vi "mini_test_app_serial_gpib (capable of overlapping tests)_qmh_ver.vi"() -> ()   [LabVIEW 2015]
doc: "This template is for the Queued Message Handler design pattern.\n\nThe Event Handling Loop generates messages based on user interface actions.\n\nThe Message Handling Loop processes messages generated by the Event Handling Loop, or by other messages. The messages are string values, so new messages can be added easily to the Message Cases case structure in the Message Handling Loop. Each message cluster can also provide an optional value for Message Data, which is a variant that can be converted to whatever message-specific data is required."
uses:
  controls/UI Data.ctl
  controls/HP Data.ctl
  Type Definitions/Highway_GB_Data.ctl
  <vilib>/Utility/error.llb/Error Cluster From Error Code.vi
  support/Message Queue/Enqueue Message (Array).vi
  support/Message Queue/Enqueue Message (Single).vi
  <vilib>/ErrorRing/Error Ring.xnode
  support/Message Queue/Message Queue.lvlib
  support/User Event - Stop/User Event - Stop.lvlib
panel:
  out "tst mod":T1(ring) caption="Test mode"
  out "GB Display":string
  out "tst time":dbl caption="total test time"
  out "overlap":dbl
  out "2d tst":dbl caption="test time 2"
  out "1st tst":dbl caption="test time 1"
  out "delay":dbl caption="delay time"
  out "GB test":dbl(slide) scale=0.0..1.0 scale format="%#_3g"
  out "HP test":dbl(slide) caption="Hi-Pot test" scale=0.0..1.0 scale format="%#_3g"
  out "HP Display":string
  out "I/F type":string caption="Interface type"
  out "GB ID":string="\r\n" caption="GB Instrument ID"
  out "HP ID":string="\r\n" caption="Hi-Pot Instrument ID"
  out "GB tst reslts":string caption="GB test results"
  out "GB tst st":string caption="GB test status"
  out "HP tst rslts":string caption="Hi-Pot test results"
  out "HP tst st":string caption="Hi-Pot test status"
  out "Display <Replace Me>":string
  in  "Stop test":bool
  in  "Start test":bool
  in  "Exit Button":bool
  # "QMH version"
  # "Hi-Pot test"
  # "GB test"
  # "Warning. This app is a proof of concept and has no other purpose, \nit is not intended for production. Use at your own risk."
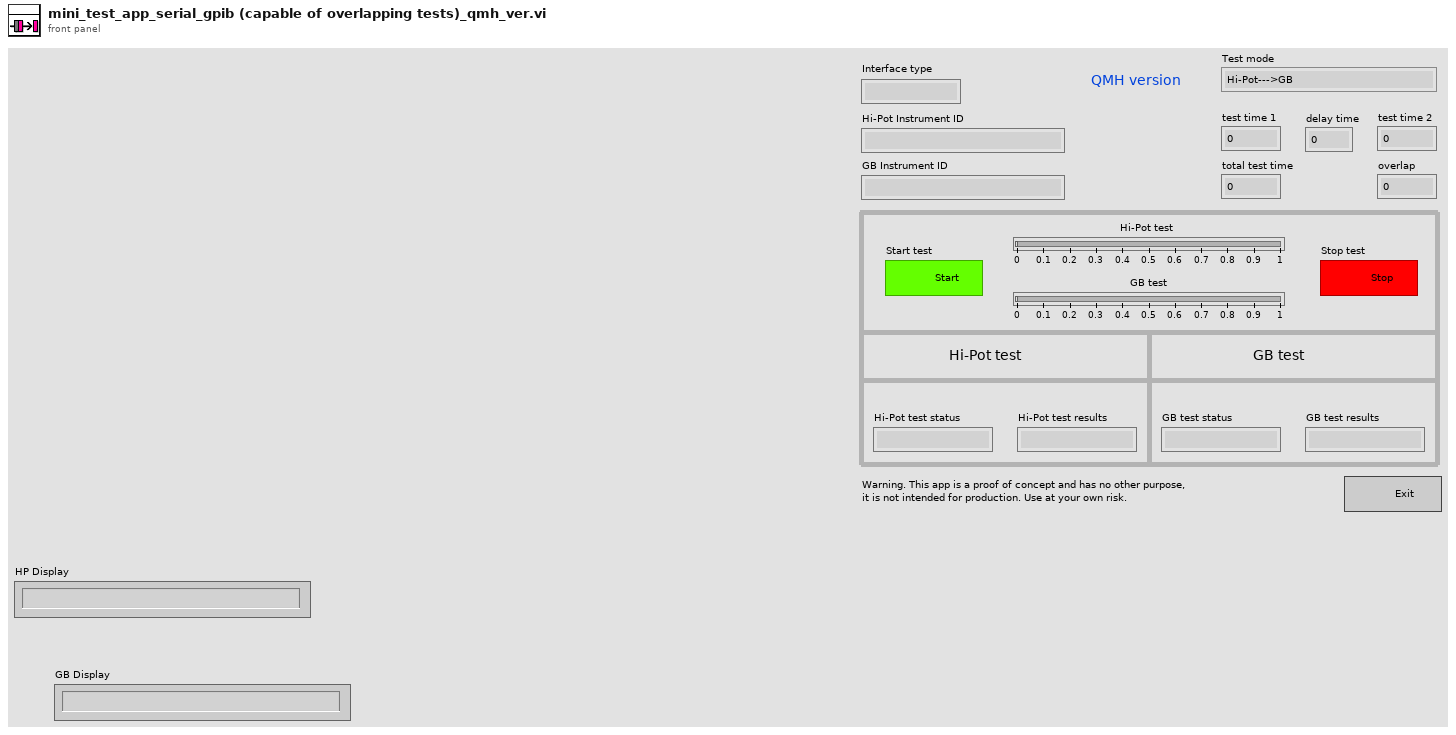
[diagram p1: front panel]
types:
  T1 = enum16{"Hi-Pot--->GB", "GB--->Hi-Pot", "Hi-Pot only", "GB only"}
  T2 = typedef "Highway_GB_Data.ctl" = cluster{"Status GB":string, "Results GB":string}
  T3 = typedef "HP Data.ctl" = cluster{"Status HP":string, "Results HP":string}
  T4 = typedef "UI Data.ctl" = cluster{"Delay Time":dbl, "prms":cluster{"1st tst":dbl, "2nd tst":dbl, "overlap":dbl, "tst time":dbl, "delay":dbl}, "test mode":enum16{"Hi-Pot--->GB", "GB--->Hi-Pot", "Hi-Pot only", "GB only"}}
  T5 = cluster{"test mode number":string, "test mode":enum16{"Hi-Pot--->GB", "GB--->Hi-Pot", "Hi-Pot only", "GB only"}, "size":i32}
  T6 = typedef "Rendezvous RefNum" = refnum<k1>
  T7 = cluster{"Rsrc name for 19572":refnum<visa-resource-name>, "Rsrc name for 19052":refnum<visa-resource-name>, "I/F type":string, "VISA2 Inst ID":string, "VISA1 Inst ID":string, "test mode":enum16{"Hi-Pot--->GB", "GB--->Hi-Pot", "Hi-Pot only", "GB only"}}
  T8 = typedef "Message Queue.lvlib/All Message Queues.ctl" = cluster{"Main":refnum<queue>, "GB Test":refnum<queue>, "HP Test":refnum<queue>}
  T9 = enum8{"Enabled", "Disabled", "Disabled and Grayed Out"}
  T10 = cluster{"1st tst":dbl, "2nd tst":dbl, "overlap":dbl, "tst time":dbl, "delay":dbl}
  T11 = cluster{"1st test":dbl, "2nd test":dbl, "overlap":dbl, "test time":dbl, "delay":dbl}
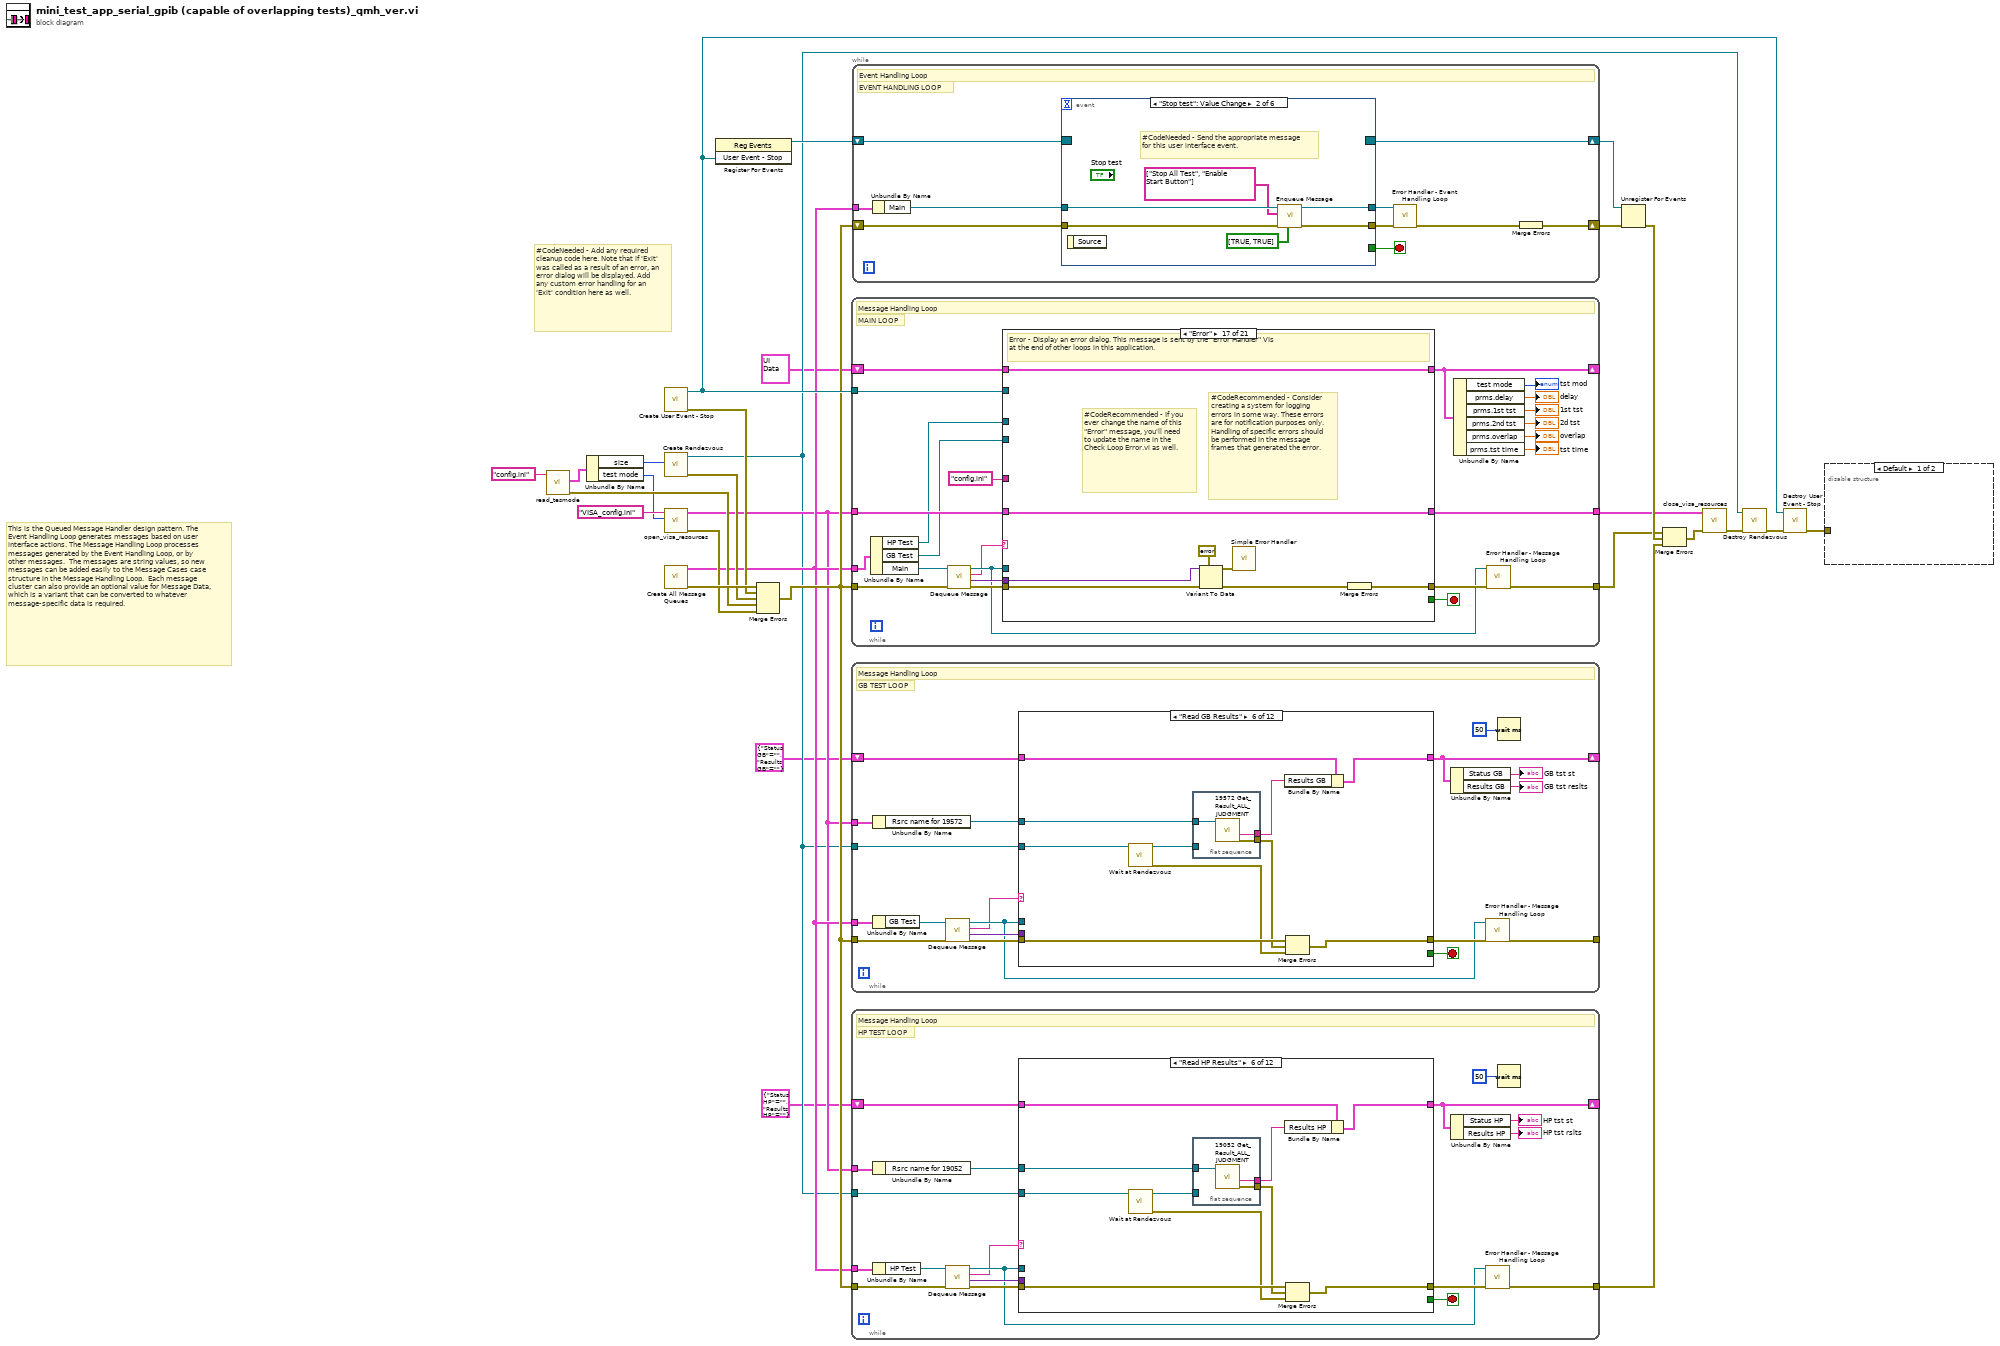
[diagram p0: block diagram]
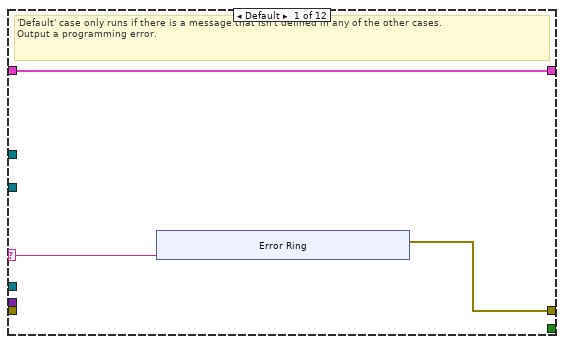
[diagram p2: hidden frame]
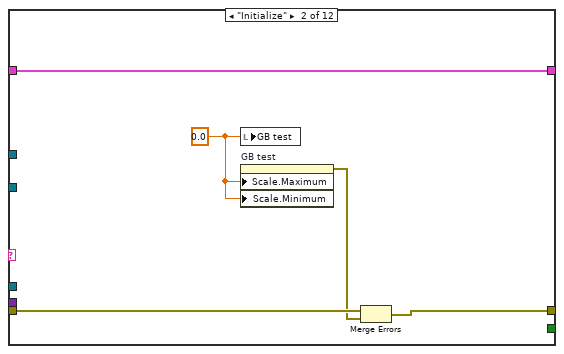
[diagram p3: hidden frame]
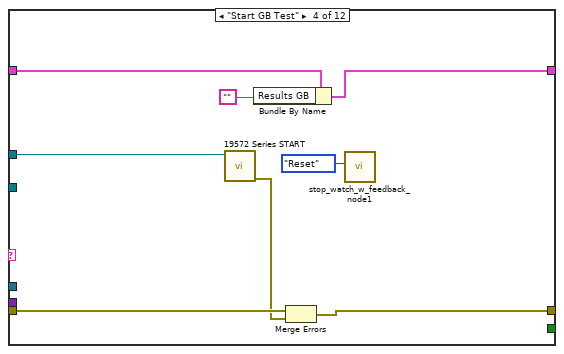
[diagram p5: hidden frame]
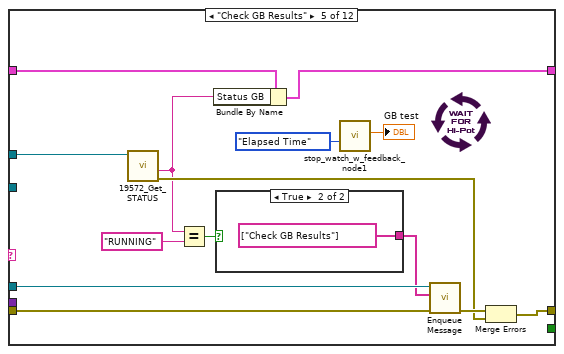
[diagram p6: hidden frame]
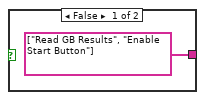
[diagram p7: hidden frame]
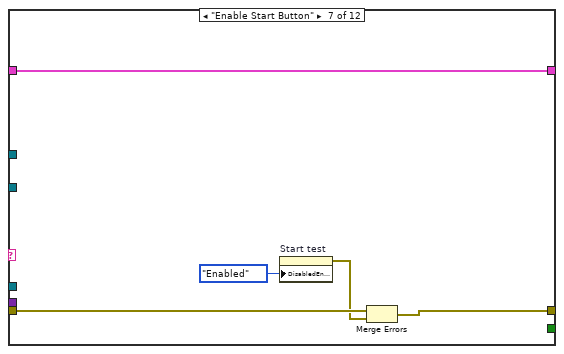
[diagram p8: hidden frame]
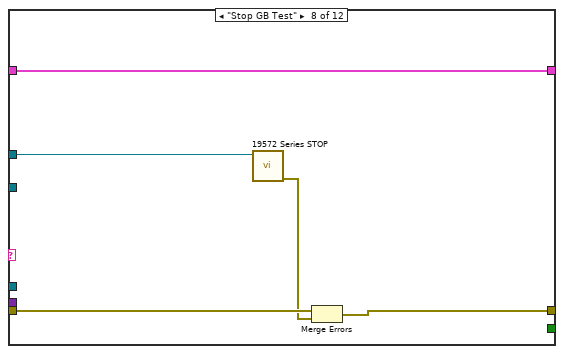
[diagram p9: hidden frame]
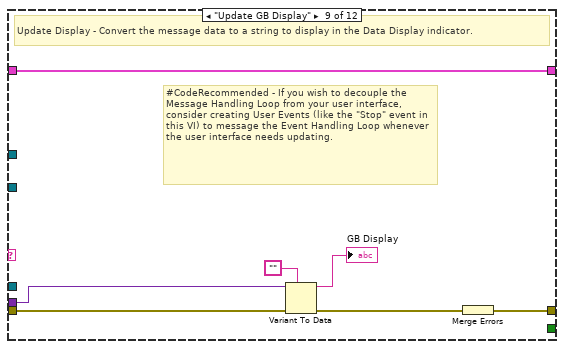
[diagram p10: hidden frame]
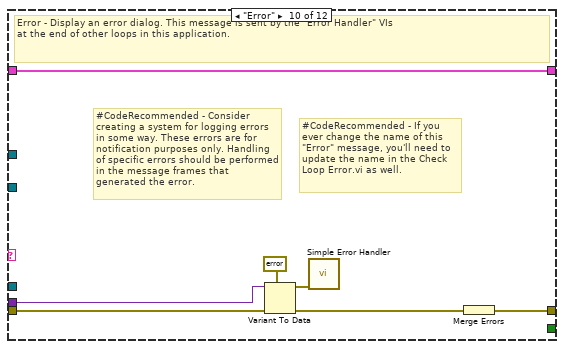
[diagram p11: hidden frame]
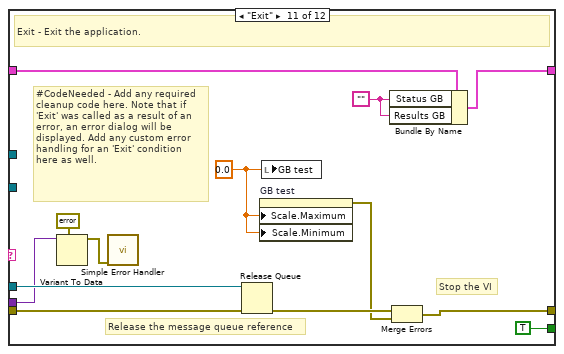
[diagram p12: hidden frame]
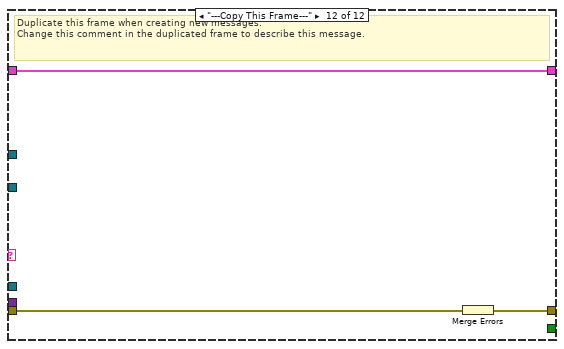
[diagram p13: hidden frame]
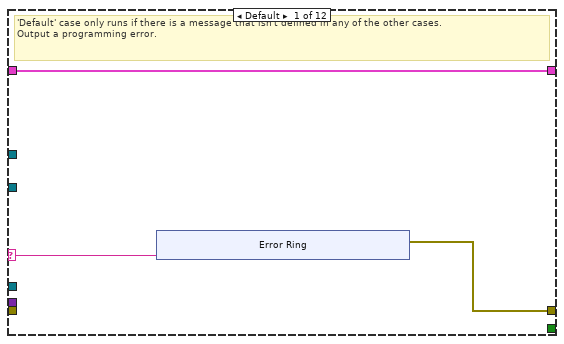
[diagram p14: hidden frame]
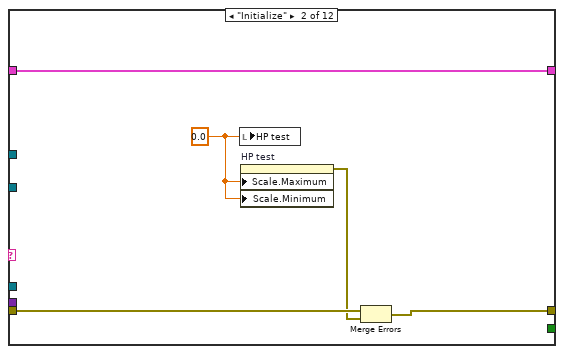
[diagram p15: hidden frame]
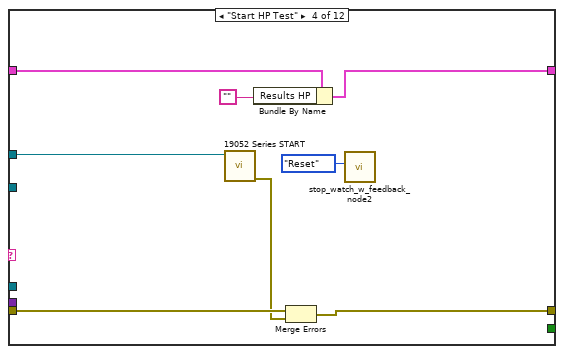
[diagram p17: hidden frame]
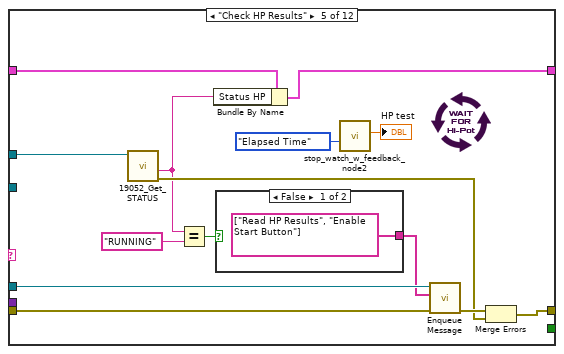
[diagram p18: hidden frame]
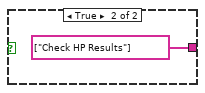
[diagram p19: hidden frame]
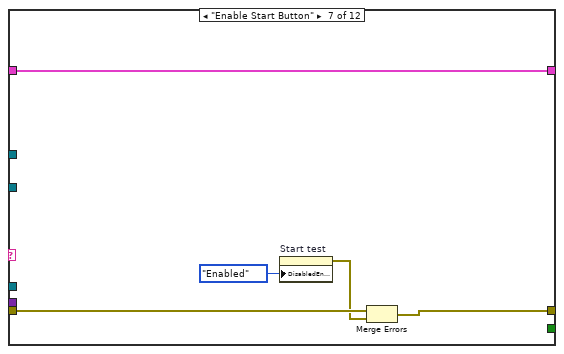
[diagram p20: hidden frame]
diagram:
  # "#CodeNeeded - Add any required cleanup code here. Note that if 'Exit' was called as a result of an error, an error dialog will be displayed. Add any custom error handling for an 'Exit' condition here as well."
  # "This is the Queued Message Handler design pattern. The Event Handling Loop generates messages based on user interface actions. The Message Handling Loop processes messages generated by the Event Handling Loop, or by other messages.  The messages are string values, so new messages can be added easily to the Message Cases case structure in the Message Handling Loop.  Each message cluster can also provide an optional value for Message Data, which is a variant that can be converted to whatever message-specific data is required."
  n1 = call "read_tesmode.vi"("config_file_name"="config.ini") -> ("error out"=w28:errorcluster, "test mode"=w6:T5)  [unwired: 8 in, 1 out]
  n2 = Unbundle By Name(w6) -> ("size"=w5:i32, "test mode"=w4:T1)
  n3 = call "Create User Event - Stop.vi"() -> ("error out"=w13:errorcluster, "User Event - Stop"=w12:refnum<user-event>)  [unwired: 10 in]
  n4 = call <vilib>:"Create Rendezvous.vi"("size (2)"=w5) -> ("error out"=w18:errorcluster, "rendezvous"=w8:T6)  [unwired: 4 in, 1 out]
  n5 = call "open_visa_resources.vi"("test mode"=w4, "config file in"="VISA_config.ini") -> ("error out"=w17:errorcluster, "VISA out"=w9:T7)  [unwired: 8 in]
  n6 = call "Create All Message Queues.vi"() -> ("error out"=w29:errorcluster, "Message Queues out"=w10:T8)  [unwired: 10 in]
  n7 = register-events(w12) -> (reference out=w24:refnum<event-registration>)  [unwired: 2 in, 1 out]
  n8 = Merge Errors(w29, w13, w18, w28, w17) -> (w11:errorcluster)
  n9 = while {
    shift-right: [w36] -> _
    shift-left: T4 {"Delay Time"=0.0, "prms"={"1st tst"=0.0, "2nd tst"=0.0, "overlap"=0.0, "tst time"=0.0, "delay"=0.0}, "test mode"=enum."Hi-Pot--->GB"} ("Data Cluster") -> [w52]
    tunnel: w12 -> [w51]
    tunnel: w11 -> [w50]
    tunnel: [w46] -> w21
    tunnel: w10 -> [w43]
    tunnel: w9 -> [w41]
    tunnel: [w40] -> w20
    stop <- w45 stop-if-true
    # "MAIN LOOP"
    # "Message Handling Loop"
    n10 = Unbundle By Name(w43) -> ("HP Test"=w39:refnum<queue>, "GB Test"=w38:refnum<queue>, "Main"=w42:refnum<queue>)
    n11 = call "Dequeue Message.vi"("error in (no error)"=w50, "Message Queue"=w42) -> ("error out"=w49:errorcluster, "Message Data"=w48:variant, "Message"=w44:string, "dup Message Queue"=w47:refnum<queue>)  [unwired: 6 in]
    n12 = case "Message Cases" shown="\"Error\"" w44 {
      selector: w44 -> [w55 _ _ _ _ _ _ _ _ _ _ _ _ _ _ _ _ _ _ _ _]
      tunnel: w47 -> [_ _ _ _ _ _ _ _ w129 _ _ _ _ _ _ _ _ w237 _ _ w270]
      tunnel: w49 -> [_ w71 w82 w92 w103 w115 w118 w124 w131 w142 w157 w171 w178 w194 w212 w218 w228 w241 w247 w255 w265]
      tunnel: [w56 w72 w81 w91 w102 w106 w118 w122 w132 w152 w167 w174 w181 w192 w208 w219 w222 w239 w245 w255 w267] -> w53
      tunnel: w52 -> [w57 w76 w80 w86 w95 w107 w117 w123 w127 w148 w163 w172 w179 w193 w211 w220 w227 w240 w246 w252 w269]
      tunnel: [w57 w76 w79 w85 w96 w107 w117 w123 w127 w148 w163 w172 w179 w193 w211 w220 w227 w240 w246 w251 w269] -> w36
      tunnel: [_ _ _ _ _ _ _ _ _ _ _ _ _ _ _ _ _ _ _ _ TRUE] -> w45
      tunnel: w48 -> [_ _ _ _ _ _ _ _ _ _ _ _ _ _ _ w217 w226 w232 _ _ w262]
      tunnel: w51 -> [_ _ _ _ _ _ _ _ _ _ _ _ _ _ _ _ _ _ _ _ w266]
      tunnel: w41 -> [w54 w74 w78 w90 w94 w114 w116 w121 w128 w151 w166 w173 w180 w187 w210 w213 w221 w236 w244 w254 w271]
      tunnel: [w54 w74 w78 w90 w94 w114 w116 w121 w128 w151 w166 w173 w180 w187 w210 w213 w221 w236 w244 w254 w271] -> w40
      tunnel: w39 -> [_ _ _ _ _ _ _ _ _ w143 w158 w168 _ w191 _ _ _ _ _ _ w258]
      tunnel: w38 -> [_ _ _ _ _ _ _ _ _ w144 w159 _ w175 w189 _ _ _ _ _ _ w257]
      tunnel: "config.ini" -> [_ _ _ w83 _ _ _ _ _ _ _ _ _ _ _ _ _ _ _ _ _]
      frame Default {
        # "'Default' case only runs if there is a message that isn't defined in any of the other cases. \nOutput a programming error."
        n13 = xnode "Error Ring"("parameter 0"=w55) -> ("error out"=w56:errorcluster)
      }
      frame "Initialize" {
        # "Bundle control references and a sample string value."
        # "Initialize - All initialization work should take place in this message, since other loops can potentially enqueue messages that execute immediately after this one."
        n14 = invoke on="Exit Button" class="Bool" method="Reinit To Default"() -> (error out=w69:errorcluster)  [unwired: 3 in, 2 out]
        n15 = invoke on="Stop test" class="Bool" method="Reinit To Default"() -> (error out=w70:errorcluster)  [unwired: 3 in, 2 out]
        n16 = Unbundle By Name(w74) -> ("VISA1 Inst ID"=→"GB ID":string, "VISA2 Inst ID"=→"HP ID":string, "I/F type"=→"I/F type":string)
        n17 = invoke on="Start test" class="Bool" method="Reinit To Default"(error in=w70) -> (error out=w68:errorcluster)  [unwired: 2 in, 2 out]
        n18 = property on="Start test" class="Bool"("DisabledEnum"=T9."Enabled" ("Disabled")) -> (error out=w67:errorcluster)  [unwired: 2 in, 1 out]
        n19 = Merge Errors(w71, w67, w69, w68) -> (w72:errorcluster)
      }
      frame "Get test mode" {
        # "Duplicate this frame when creating new messages.\nChange this comment in the duplicated frame to describe this message."
        n20 = Unbundle By Name(w78) -> ("test mode"=w77:T1)
        n21 = Merge Errors(w82) -> (w81:errorcluster)
        n22 = Bundle By Name(cluster=w80, "test mode"=w77) -> (w79:T4)
      }
      frame "Read delay time" {
        # "Duplicate this frame when creating new messages.\nChange this comment in the duplicated frame to describe this message."
        n23 = call "read_delay_time.vi"("config_file_name"=w83) -> ("error out"=w87:errorcluster, "values"=w88:cluster{"delay_time":string})  [unwired: 8 in, 1 out]
        n24 = call "delay_time_control.vi"("Higher limit"=100.0, "values in"=w88) -> ("delay time"=w84:dbl)  [unwired: 5 in]
        n25 = Merge Errors(w92, w87) -> (w91:errorcluster)
        n26 = Bundle By Name(cluster=w86, "Delay Time"=w84) -> (w85:T4)
      }
      frame "Read test params" {
        # "Duplicate this frame when creating new messages.\nChange this comment in the duplicated frame to describe this message."
        n27 = Unbundle By Name(w95) -> ("Delay Time"=w98:dbl, "test mode"=w97:T1)
        n28 = Unbundle By Name(w94) -> ("Rsrc name for 19052"=w99:refnum<visa-resource-name>, "Rsrc name for 19572"=w100:refnum<visa-resource-name>)
        n29 = call "test_definitions_module.vi"("Delay time"=w98, "VISA resource in 19572"=w100, "VISA resource in 19052"=w99, "test mode"=w97) -> ("error out"=w93:errorcluster, "Mode parameters"=w101:T11)  [unwired: 6 in]
        n30 = Bundle By Name(cluster=w95, "prms"=w101) -> (w96:T4)
        n31 = Merge Errors(w103, w93) -> (w102:errorcluster)
      }
      frame "Set Slides" {
        w113 = 0.0
        n32 = Unbundle By Name(w107) -> ("prms.1st tst"=w109:dbl, "prms.2nd tst"=w110:dbl, "test mode"=w108:T1)
        n33 = call "test_number_selector.vi"("1st tst in"=w109, "2nd tst in"=w110, "test mode"=w108) -> ("1st tst out"=w112:dbl, "2nd tst out"=w111:dbl)  [unwired: 2 in]
        n34 = property on="HP test" class="Slide (strict)"("Scale.Maximum"=w112, "Scale.Minimum"=w113) -> (error out=w104:errorcluster)  [unwired: 2 in, 1 out]
        n35 = property on="GB test" class="Slide (strict)"("Scale.Maximum"=w111, "Scale.Minimum"=w113) -> (error out=w105:errorcluster)  [unwired: 2 in, 1 out]
        n36 = Merge Errors(w115, w104, w105) -> (w106:errorcluster)
      }
      frame "Wait" {
      }
      frame "Disable Start Button" {
        # "Duplicate this frame when creating new messages.\nChange this comment in the duplicated frame to describe this message."
        n37 = property on="Start test" class="Bool"("DisabledEnum"=T9."Disabled and Grayed Out" ("Disabled")) -> (error out=w119:errorcluster)  [unwired: 2 in, 1 out]
        n38 = Merge Errors(w124, w119) -> (w122:errorcluster)
      }
      frame "Check Test Mode" {
        # "Send string to \"Update Display\" message"
        # "#CodeNeeded - Perform whatever actions correspond to the \"Something\" message."
        # "Something - Replace this message with functionality for your own application."
        n39 = Unbundle By Name(w127) -> ("test mode"=w126:T1)
        n40 = case shown="\"GB--->Hi-Pot\"" w126 {
          tunnel: ["Wait" "Start HP-->GB" "Start GB-->HP" "Start HP only" "Start GB only"] -> w125
          frame Default {
          }
          frame "Hi-Pot--->GB" {
          }
          frame "GB--->Hi-Pot" {
          }
          frame "Hi-Pot only" {
          }
          frame "GB only" {
          }
        }
        n41 = call-poly "Enqueue Message.vi"("error in (no error)"=w131, "Message"=w125, "Message Queue"=w129) -> ("error out"=w130:errorcluster)  [unwired: 7 in, 1 out]
        n42 = Merge Errors(w130) -> (w132:errorcluster)
      }
      frame "Start HP-->GB" {
        # "#CodeNeeded - Perform whatever actions correspond to the \"Something Else\" message."
        # "Something Else - Replace this message with functionality for your own application."
        n43 = call "select_queue_path.vi"("Control"=enum16{"Invert", "Direct"}."Invert", "Message Queue 2"=w144, "Message Queue"=w143) -> ("dup Message Queue 2"=w146:refnum<queue>, "dup Message Queue"=w145:refnum<queue>)  [unwired: 7 in]
        n44 = Unbundle By Name(w148) -> ("prms.delay"=w138:dbl)
        n45 = call-poly "Enqueue Message.vi"("Message Array"=string[] ["Start HP Test", "Check HP Results"], "Message Queue"=w146) -> ("error out"=w150:errorcluster)  [unwired: 8 in, 1 out]
        n46 = call "Time Delay"("error in (no error)"=w150, "Delay Time (s)"=w138) -> ("error out"=w149:errorcluster)  [unwired: 9 in]
        n47 = call-poly "Enqueue Message.vi"("error in (no error)"=w149, "Message Array"=string[] ["Start GB Test", "Check GB Results"], "Message Queue"=w145) -> ("error out"=w141:errorcluster)  [unwired: 7 in, 1 out]
        n48 = Merge Errors(w142, w141) -> (w152:errorcluster)
      }
      frame "Start GB-->HP" {
        # "#CodeNeeded - Perform whatever actions correspond to the \"Something Else\" message."
        # "Something Else - Replace this message with functionality for your own application."
        n49 = call "select_queue_path.vi"("Control"=enum16{"Invert", "Direct"}."Direct", "Message Queue 2"=w159, "Message Queue"=w158) -> ("dup Message Queue 2"=w161:refnum<queue>, "dup Message Queue"=w160:refnum<queue>)  [unwired: 7 in]
        n50 = Unbundle By Name(w163) -> ("prms.delay"=w153:dbl)
        n51 = call-poly "Enqueue Message.vi"("Message Array"=string[] ["Start GB Test", "Check GB Results"], "Message Queue"=w161) -> ("error out"=w165:errorcluster)  [unwired: 8 in, 1 out]
        n52 = call "Time Delay2"("error in (no error)"=w165, "Delay Time (s)"=w153) -> ("error out"=w164:errorcluster)  [unwired: 9 in]
        n53 = call-poly "Enqueue Message.vi"("error in (no error)"=w164, "Message Array"=string[] ["Start HP Test", "Check HP Results"], "Message Queue"=w160) -> ("error out"=w156:errorcluster)  [unwired: 7 in, 1 out]
        n54 = Merge Errors(w157, w156) -> (w167:errorcluster)
      }
      frame "Start HP only" {
        # "#CodeNeeded - Perform whatever actions correspond to the \"Something Else\" message."
        # "Something Else - Replace this message with functionality for your own application."
        n55 = call-poly "Enqueue Message.vi"("Message Array"=string[] ["Start HP Test", "Check HP Results"], "Message Queue"=w168) -> ("error out"=w170:errorcluster)  [unwired: 8 in, 1 out]
        n56 = Merge Errors(w171, w170) -> (w174:errorcluster)
      }
      frame "Start GB only" {
        # "#CodeNeeded - Perform whatever actions correspond to the \"Something Else\" message."
        # "Something Else - Replace this message with functionality for your own application."
        n57 = call-poly "Enqueue Message.vi"("Message Array"=string[] ["Start GB Test", "Check GB Results"], "Message Queue"=w175) -> ("error out"=w177:errorcluster)  [unwired: 8 in, 1 out]
        n58 = Merge Errors(w178, w177) -> (w181:errorcluster)
      }
      frame "Stop All Test" {
        n59 = Unbundle By Name(w187) -> ("test mode"=w186:T1)
        n60 = case shown="\"GB only\"" w186 {
          tunnel: w191 -> [w197 w202 w206]
          tunnel: [w197 w202 w206] -> w190
          tunnel: w189 -> [w196 w201 w205]
          tunnel: [w196 w201 w205] -> w188
          tunnel: ["Wait" "Stop GB Test" "Stop GB Test"] -> w185
          tunnel: ["Stop HP Test" "Stop HP Test" "Wait"] -> w184
          frame "Hi-Pot only" {
          }
          frame "Hi-Pot--->GB", "GB--->Hi-Pot" {
          }
          frame "GB only" {
          }
        }
        n61 = call-poly "Enqueue Message.vi"("Message"=w185, "Message Queue"=w188) -> ("error out"=w182:errorcluster)  [unwired: 8 in, 1 out]
        n62 = call-poly "Enqueue Message.vi"("Message"=w184, "Message Queue"=w190) -> ("error out"=w183:errorcluster)  [unwired: 8 in, 1 out]
        n63 = Merge Errors(w194, w183, w182) -> (w192:errorcluster)
      }
      frame "Enable Start Button" {
        n64 = property on="Start test" class="Bool"("DisabledEnum"=T9."Enabled" ("Disabled")) -> (error out=w207:errorcluster)  [unwired: 2 in, 1 out]
        n65 = Merge Errors(w212, w207) -> (w208:errorcluster)
      }
      frame "Update Display" {
        # "#CodeRecommended - If you wish to decouple the Message Handling Loop from your user interface, consider creating User Events (like the \"Stop\" event in this VI) to message the Event Handling Loop whenever the user interface needs updating."
        # "Update Display - Convert the message data to a string to display in the Data Display indicator."
        n66 = Variant To Data(error in=w218, type="", Variant=w217) -> (data=→"Display <Replace Me>":string, error out=w215:errorcluster)
        n67 = Merge Errors(w215) -> (w219:errorcluster)
      }
      frame "Error" {
        # "#CodeRecommended - If you ever change the name of this \"Error\" message, you'll need to update the name in the Check Loop Error.vi as well."
        # "#CodeRecommended - Consider creating a system for logging errors in some way. These errors are for notification purposes only. Handling of specific errors should be performed in the message frames that generated the error."
        # "Error - Display an error dialog. This message is sent by the \"Error Handler\" VIs \nat the end of other loops in this application."
        n68 = Variant To Data(error in=w228, type=errorcluster {"status"=FALSE, "code"=0, "source"=""} ("error constant"), Variant=w226) -> (data=w224:errorcluster, error out=w223:errorcluster)
        n69 = call <vilib>:"Simple Error Handler.vi"("error in (no error)"=w224) -> ()  [unwired: 4 in, 5 out]
        n70 = Merge Errors(w223) -> (w222:errorcluster)
      }
      frame "Confirm Quit" {
        # "#CodeNeeded - If you want to provide an \"Are you sure\" dialog (or some other notification) before the application exits, place that code here. This message is typically sent from a Panel Close? event."
        # "Confirm Quit - Message that can confirm whether or not the user wants to exit the application."
        n71 = Variant To Data(type="", Variant=w232) -> (data=w231:string, error out=w230:errorcluster)  [unwired: 1 in]
        n72 = Two Button Dialog(message=w231) -> (T button?=w235:bool)  [unwired: 2 in]
        n73 = case shown="True" w235 {
          tunnel: [string[] ["Wait"] string[] ["Exit", "Turn Off Indicators"]] -> w229
          frame False {
          }
          frame True {
          }
        }
        n74 = call-poly "Enqueue Message.vi"("Priority Message? Array"=bool[] [TRUE, TRUE], "error in (no error)"=w241, "Message Array"=w229, "Message Queue"=w237) -> ("error out"=w238:errorcluster)  [unwired: 6 in, 1 out]
        n75 = Merge Errors(w238, w230) -> (w239:errorcluster)
      }
      frame "---Copy This Frame---" {
        # "Duplicate this frame when creating new messages. Change this comment in the duplicated frame to describe this message."
        n76 = Merge Errors(w247) -> (w245:errorcluster)
      }
      frame "Turn Off Indicators" {
        w250 = ""
        n77 = local write "I/F type"(w250) -> ()
        n78 = local write "HP ID"(w250) -> ()
        n79 = local write "GB ID"(w250) -> ()
        n80 = Bundle By Name(cluster=w252, "test mode"=T1."Hi-Pot only", "Delay Time"=0.0, "prms"=T10 {"1st tst"=0.0, "2nd tst"=0.0, "overlap"=0.0, "tst time"=0.0, "delay"=0.0}) -> (w251:T4)
      }
      frame "Exit" {
        # "Stop the VI"
        # "Release the message queue reference"
        # "Exit - Exit the application."
        n81 = Variant To Data(type=errorcluster {"status"=FALSE, "code"=0, "source"=""} ("error constant"), Variant=w262) -> (data=w263:errorcluster)  [unwired: 1 in, 1 out]
        n82 = call <vilib>:"Simple Error Handler.vi"("error in (no error)"=w263) -> ()  [unwired: 4 in, 5 out]
        n83 = Unbundle By Name(w271) -> ("test mode"=w256:T1)
        n84 = Release Queue(queue=w270, error in (no error)=w265) -> (error out=w261:errorcluster)  [unwired: 1 in, 2 out]
        n85 = call "exit-tasks.vi"("test mode"=w256, "GB Test Queue"=w257, "HP Test Queue"=w258) -> ("error out"=w259:errorcluster)  [unwired: 8 in]
        n86 = call "Fire User Event - Stop.vi"("User Event - Stop"=w266) -> ("error out"=w260:errorcluster)  [unwired: 10 in]
        n87 = Merge Errors(w261, w260, w259) -> (w267:errorcluster)
      }
    }
    n88 = Unbundle By Name(w36) -> ("test mode"=→"tst mod":T1, "prms.delay"=→"delay":dbl, "prms.1st tst"=→"1st tst":dbl, "prms.2nd tst"=→"2d tst":dbl, "prms.overlap"=→"overlap":dbl, "prms.tst time"=→"tst time":dbl)
    n89 = call "Error Handler - Message Handling Loop.vi"("error in (no error)"=w53, "Message Queue"=w47) -> ("dup error in"=w46:errorcluster)  [unwired: 8 in, 1 out]
  }
  n90 = while {
    shift-right: [w279] -> _
    shift-left: T2 {"Status GB"="", "Results GB"=""} ("Data Cluster") -> [w288]
    tunnel: w11 -> [w287]
    tunnel: [w283] -> _
    tunnel: w9 -> [w281]
    tunnel: w10 -> [w277]
    tunnel: w8 -> [w275]
    stop <- w282 stop-if-true
    # "GB TEST LOOP"
    # "Message Handling Loop"
    n91 = Unbundle By Name(w281) -> ("Rsrc name for 19572"=w280:refnum<visa-resource-name>)
    n92 = Unbundle By Name(w277) -> ("GB Test"=w276:refnum<queue>)
    n93 = call "Dequeue Message.vi"("error in (no error)"=w287, "Message Queue"=w276) -> ("error out"=w286:errorcluster, "Message Data"=w285:variant, "Message"=w274:string, "dup Message Queue"=w284:refnum<queue>)  [unwired: 6 in]
    n94 = case "Message Cases" shown="\"Read GB Results\"" w274 {
      selector: w274 -> [w290 _ _ _ _ _ _ _ _ _ _ _]
      tunnel: w284 -> [_ _ _ _ w325 _ _ _ _ _ w380 _]
      tunnel: w286 -> [_ w302 w306 w313 w327 w340 w348 w350 w358 w367 w376 w383]
      tunnel: [w291 w301 w306 w312 w328 w339 w345 w352 w359 w361 w377 w381] -> w289
      tunnel: w288 -> [w292 w304 w305 w309 w323 w336 w347 w353 w360 w366 w370 w382]
      tunnel: [w292 w304 w305 w308 w322 w335 w347 w353 w360 w366 w369 w382] -> w279
      tunnel: [_ _ _ _ _ _ _ _ _ _ TRUE _] -> w282
      tunnel: w285 -> [_ _ _ _ _ _ _ _ w357 w365 w373 _]
      tunnel: w280 -> [_ _ _ w314 w324 w338 _ w351 _ _ _ _]
      tunnel: w275 -> [_ _ _ _ _ w331 _ _ _ _ _ _]
      frame Default {
        # "'Default' case only runs if there is a message that isn't defined in any of the other cases. \nOutput a programming error."
        n95 = xnode "Error Ring"("parameter 0"=w290) -> ("error out"=w291:errorcluster)
      }
      frame "Initialize" {
        w303 = 0.0
        n96 = local write "GB test"(w303) -> ()
        n97 = property on="GB test" class="Slide (strict)"("Scale.Maximum"=w303, "Scale.Minimum"=w303) -> (error out=w300:errorcluster)  [unwired: 2 in, 1 out]
        n98 = Merge Errors(w302, w300) -> (w301:errorcluster)
      }
      frame "Wait" {
      }
      frame "Start GB Test" {
        n99 = call "19572 Series START.vi"("VISA resource in"=w314) -> ("error out"=w311:errorcluster)  [unwired: 9 in, 1 out]
        n100 = Bundle By Name(cluster=w309, "Results GB"="") -> (w308:T2)
        n101 = Merge Errors(w313, w311) -> (w312:errorcluster)
        n102 = call "stop_watch_w_feedback_node1.vi"("Command"=enum16{"Elapsed Time", "Reset"}."Reset") -> ()  [unwired: 10 in, 1 out]
      }
      frame "Check GB Results" {
        n103 = call "19572_Get_STATUS.vi"("VISA resource in"=w324) -> ("error out"=w318:errorcluster, "Status"=w317:string)  [unwired: 8 in, 1 out]
        n104 = Equal?(x=w317, y="RUNNING") -> (x = y?=w320:bool)
        n105 = Bundle By Name(cluster=w323, "Status GB"=w317) -> (w322:T2)
        n106 = case shown="True" w320 {
          tunnel: [string[] ["Read GB Results", "Enable Start Button"] string[] ["Check GB Results"]] -> w319
          frame False {
          }
          frame True {
          }
        }
        n107 = call "stop_watch_w_feedback_node1.vi"("Command"=enum16{"Elapsed Time", "Reset"}."Elapsed Time") -> ("Elapsed Time"=→"GB test":dbl)  [unwired: 10 in]
        n108 = call-poly "Enqueue Message.vi"("error in (no error)"=w327, "Message Array"=w319, "Message Queue"=w325) -> ("error out"=w326:errorcluster)  [unwired: 7 in, 1 out]
        n109 = Merge Errors(w326, w318) -> (w328:errorcluster)
      }
      frame "Read GB Results" {
        n110 = call <vilib>:"Wait at Rendezvous.vi"("rendezvous"=w331) -> ("error out"=w332:errorcluster, "rendezvous out"=w333:T6)  [unwired: 4 in, 1 out]
        n111 = flat-sequence {
          tunnel: w338 -> [w343]
          tunnel: [w342] -> w337
          tunnel: [w341] -> w334
          tunnel: w333 -> [_]
          frame #0 {
            n112 = call "19572 Get_Result_ALL_JUDGMENT.vi"("VISA resource in"=w343) -> ("error out"=w342:errorcluster, "JUDGMENT"=w341:string)  [unwired: 8 in, 1 out]
          }
        }
        n113 = Bundle By Name(cluster=w336, "Results GB"=w334) -> (w335:T2)
        n114 = Merge Errors(w340, w337, w332) -> (w339:errorcluster)
      }
      frame "Enable Start Button" {
        n115 = property on="Start test" class="Bool"("DisabledEnum"=T9."Enabled" ("Disabled")) -> (error out=w344:errorcluster)  [unwired: 2 in, 1 out]
        n116 = Merge Errors(w348, w344) -> (w345:errorcluster)
      }
      frame "Stop GB Test" {
        n117 = call "19572 Series STOP.vi"("VISA resource in"=w351) -> ("error out"=w349:errorcluster)  [unwired: 9 in, 1 out]
        n118 = Merge Errors(w350, w349) -> (w352:errorcluster)
      }
      frame "Update GB Display" {
        # "#CodeRecommended - If you wish to decouple the Message Handling Loop from your user interface, consider creating User Events (like the \"Stop\" event in this VI) to message the Event Handling Loop whenever the user interface needs updating."
        # "Update Display - Convert the message data to a string to display in the Data Display indicator."
        n119 = Variant To Data(error in=w358, type="", Variant=w357) -> (data=→"GB Display":string, error out=w355:errorcluster)
        n120 = Merge Errors(w355) -> (w359:errorcluster)
      }
      frame "Error" {
        # "#CodeRecommended - If you ever change the name of this \"Error\" message, you'll need to update the name in the Check Loop Error.vi as well."
        # "#CodeRecommended - Consider creating a system for logging errors in some way. These errors are for notification purposes only. Handling of specific errors should be performed in the message frames that generated the error."
        # "Error - Display an error dialog. This message is sent by the \"Error Handler\" VIs \nat the end of other loops in this application."
        n121 = Variant To Data(error in=w367, type=errorcluster {"status"=FALSE, "code"=0, "source"=""} ("error constant"), Variant=w365) -> (data=w363:errorcluster, error out=w362:errorcluster)
        n122 = call <vilib>:"Simple Error Handler.vi"("error in (no error)"=w363) -> ()  [unwired: 4 in, 5 out]
        n123 = Merge Errors(w362) -> (w361:errorcluster)
      }
      frame "Exit" {
        w368 = ""
        w372 = 0.0 ("HP test")
        # "Stop the VI"
        # "Release the message queue reference"
        # "#CodeNeeded - Add any required cleanup code here. Note that if 'Exit' was called as a result of an error, an error dialog will be displayed. Add any custom error handling for an 'Exit' condition here as well."
        # "Exit - Exit the application."
        n124 = Variant To Data(type=errorcluster {"status"=FALSE, "code"=0, "source"=""} ("error constant"), Variant=w373) -> (data=w374:errorcluster)  [unwired: 1 in, 1 out]
        n125 = call <vilib>:"Simple Error Handler.vi"("error in (no error)"=w374) -> ()  [unwired: 4 in, 5 out]
        n126 = Release Queue(queue=w380, error in (no error)=w376) -> (error out=w378:errorcluster)  [unwired: 1 in, 2 out]
        n127 = property on="GB test" class="Slide (strict)"("Scale.Maximum"=w372, "Scale.Minimum"=w372) -> (error out=w371:errorcluster)  [unwired: 2 in, 1 out]
        n128 = local write "GB test"(w372) -> ()
        n129 = Bundle By Name(cluster=w370, "Status GB"=w368, "Results GB"=w368) -> (w369:T2)
        n130 = Merge Errors(w378, w371) -> (w377:errorcluster)
      }
      frame "---Copy This Frame---" {
        # "Duplicate this frame when creating new messages.\nChange this comment in the duplicated frame to describe this message."
        n131 = Merge Errors(w383) -> (w381:errorcluster)
      }
    }
    n132 = Unbundle By Name(w279) -> ("Status GB"=→"GB tst st":string, "Results GB"=→"GB tst reslts":string)
    n133 = call "Error Handler - Message Handling Loop.vi"("error in (no error)"=w289, "Message Queue"=w284) -> ("dup error in"=w283:errorcluster)  [unwired: 8 in, 1 out]
    n134 = Wait (ms)(milliseconds to wait=u32 50) -> ()  [unwired: 1 out]
  }
  n135 = while {
    shift-right: [w391] -> _
    shift-left: T3 {"Status HP"="", "Results HP"=""} ("Data Cluster") -> [w400]
    tunnel: w11 -> [w399]
    tunnel: [w395] -> w23
    tunnel: w9 -> [w393]
    tunnel: w10 -> [w387]
    tunnel: w8 -> [w385]
    stop <- w394 stop-if-true
    # "HP TEST LOOP"
    # "Message Handling Loop"
    n136 = Unbundle By Name(w393) -> ("Rsrc name for 19052"=w392:refnum<visa-resource-name>)
    n137 = Unbundle By Name(w387) -> ("HP Test"=w386:refnum<queue>)
    n138 = call "Dequeue Message.vi"("error in (no error)"=w399, "Message Queue"=w386) -> ("error out"=w398:errorcluster, "Message Data"=w397:variant, "Message"=w384:string, "dup Message Queue"=w396:refnum<queue>)  [unwired: 6 in]
    n139 = case "Message Cases" shown="\"Read HP Results\"" w384 {
      selector: w384 -> [w402 _ _ _ _ _ _ _ _ _ _ _]
      tunnel: w396 -> [_ _ _ _ w437 _ _ _ _ _ w492 _]
      tunnel: w398 -> [_ w414 w418 w425 w439 w452 w460 w462 w470 w479 w488 w495]
      tunnel: [w403 w413 w418 w424 w440 w451 w457 w464 w471 w473 w489 w493] -> w401
      tunnel: w400 -> [w404 w416 w417 w421 w435 w448 w459 w465 w472 w478 w482 w494]
      tunnel: [w404 w416 w417 w420 w434 w447 w459 w465 w472 w478 w481 w494] -> w391
      tunnel: [_ _ _ _ _ _ _ _ _ _ TRUE _] -> w394
      tunnel: w397 -> [_ _ _ _ _ _ _ _ w469 w477 w485 _]
      tunnel: w392 -> [_ _ _ w426 w436 w450 _ w463 _ _ _ _]
      tunnel: w385 -> [_ _ _ _ _ w443 _ _ _ _ _ _]
      frame Default {
        # "'Default' case only runs if there is a message that isn't defined in any of the other cases. \nOutput a programming error."
        n140 = xnode "Error Ring"("parameter 0"=w402) -> ("error out"=w403:errorcluster)
      }
      frame "Initialize" {
        w415 = 0.0
        n141 = local write "HP test"(w415) -> ()
        n142 = property on="HP test" class="Slide (strict)"("Scale.Maximum"=w415, "Scale.Minimum"=w415) -> (error out=w412:errorcluster)  [unwired: 2 in, 1 out]
        n143 = Merge Errors(w414, w412) -> (w413:errorcluster)
      }
      frame "Wait" {
      }
      frame "Start HP Test" {
        n144 = call "19052 Series START.vi"("VISA resource in"=w426) -> ("error out"=w423:errorcluster)  [unwired: 9 in, 1 out]
        n145 = Bundle By Name(cluster=w421, "Results HP"="") -> (w420:T3)
        n146 = Merge Errors(w425, w423) -> (w424:errorcluster)
        n147 = call "stop_watch_w_feedback_node2.vi"("Command"=enum16{"Elapsed Time", "Reset"}."Reset") -> ()  [unwired: 10 in, 1 out]
      }
      frame "Check HP Results" {
        n148 = call "19052_Get_STATUS.vi"("VISA resource in"=w436) -> ("error out"=w430:errorcluster, "Status"=w429:string)  [unwired: 8 in, 1 out]
        n149 = Equal?(x=w429, y="RUNNING") -> (x = y?=w432:bool)
        n150 = Bundle By Name(cluster=w435, "Status HP"=w429) -> (w434:T3)
        n151 = case shown="False" w432 {
          tunnel: [string[] ["Read HP Results", "Enable Start Button"] string[] ["Check HP Results"]] -> w431
          frame False {
          }
          frame True {
          }
        }
        n152 = call "stop_watch_w_feedback_node2.vi"("Command"=enum16{"Elapsed Time", "Reset"}."Elapsed Time") -> ("Elapsed Time"=→"HP test":dbl)  [unwired: 10 in]
        n153 = call-poly "Enqueue Message.vi"("error in (no error)"=w439, "Message Array"=w431, "Message Queue"=w437) -> ("error out"=w438:errorcluster)  [unwired: 7 in, 1 out]
        n154 = Merge Errors(w438, w430) -> (w440:errorcluster)
      }
      frame "Read HP Results" {
        n155 = call <vilib>:"Wait at Rendezvous.vi"("rendezvous"=w443) -> ("error out"=w444:errorcluster, "rendezvous out"=w445:T6)  [unwired: 4 in, 1 out]
        n156 = flat-sequence {
          tunnel: w450 -> [w455]
          tunnel: [w454] -> w449
          tunnel: [w453] -> w446
          tunnel: w445 -> [_]
          frame #0 {
            n157 = call "19052 Get_Result_ALL_JUDGMENT.vi"("VISA resource in"=w455) -> ("error out"=w454:errorcluster, "JUDGMENT"=w453:string)  [unwired: 8 in, 1 out]
          }
        }
        n158 = Bundle By Name(cluster=w448, "Results HP"=w446) -> (w447:T3)
        n159 = Merge Errors(w452, w449, w444) -> (w451:errorcluster)
      }
      frame "Enable Start Button" {
        n160 = property on="Start test" class="Bool"("DisabledEnum"=T9."Enabled" ("Disabled")) -> (error out=w456:errorcluster)  [unwired: 2 in, 1 out]
        n161 = Merge Errors(w460, w456) -> (w457:errorcluster)
      }
      frame "Stop HP Test" {
        n162 = call "19052 Series STOP.vi"("VISA resource in"=w463) -> ("error out"=w461:errorcluster)  [unwired: 9 in, 1 out]
        n163 = Merge Errors(w462, w461) -> (w464:errorcluster)
      }
      frame "Update HP Display" {
        # "#CodeRecommended - If you wish to decouple the Message Handling Loop from your user interface, consider creating User Events (like the \"Stop\" event in this VI) to message the Event Handling Loop whenever the user interface needs updating."
        # "Update Display - Convert the message data to a string to display in the Data Display indicator."
        n164 = Variant To Data(error in=w470, type="", Variant=w469) -> (data=→"HP Display":string, error out=w467:errorcluster)
        n165 = Merge Errors(w467) -> (w471:errorcluster)
      }
      frame "Error" {
        # "#CodeRecommended - If you ever change the name of this \"Error\" message, you'll need to update the name in the Check Loop Error.vi as well."
        # "#CodeRecommended - Consider creating a system for logging errors in some way. These errors are for notification purposes only. Handling of specific errors should be performed in the message frames that generated the error."
        # "Error - Display an error dialog. This message is sent by the \"Error Handler\" VIs \nat the end of other loops in this application."
        n166 = Variant To Data(error in=w479, type=errorcluster {"status"=FALSE, "code"=0, "source"=""} ("error constant"), Variant=w477) -> (data=w475:errorcluster, error out=w474:errorcluster)
        n167 = call <vilib>:"Simple Error Handler.vi"("error in (no error)"=w475) -> ()  [unwired: 4 in, 5 out]
        n168 = Merge Errors(w474) -> (w473:errorcluster)
      }
      frame "Exit" {
        w480 = ""
        w484 = 0.0 ("HP test")
        # "Stop the VI"
        # "Release the message queue reference"
        # "#CodeNeeded - Add any required cleanup code here. Note that if 'Exit' was called as a result of an error, an error dialog will be displayed. Add any custom error handling for an 'Exit' condition here as well."
        # "Exit - Exit the application."
        n169 = Variant To Data(type=errorcluster {"status"=FALSE, "code"=0, "source"=""} ("error constant"), Variant=w485) -> (data=w486:errorcluster)  [unwired: 1 in, 1 out]
        n170 = call <vilib>:"Simple Error Handler.vi"("error in (no error)"=w486) -> ()  [unwired: 4 in, 5 out]
        n171 = Release Queue(queue=w492, error in (no error)=w488) -> (error out=w490:errorcluster)  [unwired: 1 in, 2 out]
        n172 = property on="HP test" class="Slide (strict)"("Scale.Maximum"=w484, "Scale.Minimum"=w484) -> (error out=w483:errorcluster)  [unwired: 2 in, 1 out]
        n173 = local write "HP test"(w484) -> ()
        n174 = Bundle By Name(cluster=w482, "Status HP"=w480, "Results HP"=w480) -> (w481:T3)
        n175 = Merge Errors(w490, w483) -> (w489:errorcluster)
      }
      frame "---Copy This Frame---" {
        # "Duplicate this frame when creating new messages.\nChange this comment in the duplicated frame to describe this message."
        n176 = Merge Errors(w495) -> (w493:errorcluster)
      }
    }
    n177 = Unbundle By Name(w391) -> ("Status HP"=→"HP tst st":string, "Results HP"=→"HP tst rslts":string)
    n178 = call "Error Handler - Message Handling Loop.vi"("error in (no error)"=w401, "Message Queue"=w396) -> ("dup error in"=w395:errorcluster)  [unwired: 8 in, 1 out]
    n179 = Wait (ms)(milliseconds to wait=u32 50) -> ()  [unwired: 1 out]
  }
  n180 = while {
    shift-right: [w504] -> w26
    shift-left: w24 -> [w505]
    tunnel: w10 -> [w498]
    shift-right: [w499] -> w25
    shift-left: w11 -> [w496]
    stop <- w502 stop-if-true
    # "EVENT HANDLING LOOP"
    # "Event Handling Loop"
    n181 = Unbundle By Name(w498) -> ("Main"=w497:refnum<queue>)
    n182 = event shown="[1] \"Stop test\": Value Change" {
      selector: w505 -> [_ _ _ _ _ _]
      dyn-events: [_ _ _ _ _ _] -> w504
      timeout: _ -> [_ _ _ _ _ _]
      tunnel: [_ _ _ _ _ TRUE ("Discard?")] -> w502
      tunnel: w497 -> [w510 w516 w523 w526 w532 w536]
      tunnel: [w507 w513 w522 w525 w529 w533] -> w503
      tunnel: [w509 w515 w521 w526 w531 w536] -> w501
      tunnel: w496 -> [w508 w514 w520 w525 w530 w533]
      event "Start test": Value Change {
        # "#CodeNeeded - Send the appropriate message for this user interface event."
        n183 = event-data() -> ()  [unwired: 1 in, 1 out]
        n184 = call-poly "Enqueue Message.vi"("error in (no error)"=w508, "Message Array"=string[] ["Disable Start Button", "Check Test Mode"], "Message Queue"=w510) -> ("error out"=w507:errorcluster, "dup Message Queue"=w509:refnum<queue>)  [unwired: 7 in]
      }
      event "Stop test": Value Change {
        # "#CodeNeeded - Send the appropriate message for this user interface event."
        n185 = event-data() -> ()  [unwired: 1 in, 1 out]
        n186 = call-poly "Enqueue Message.vi"("Priority Message? Array"=bool[] [TRUE, TRUE], "error in (no error)"=w514, "Message Array"=string[] ["Stop All Test", "Enable Start Button"], "Message Queue"=w516) -> ("error out"=w513:errorcluster, "dup Message Queue"=w515:refnum<queue>)  [unwired: 6 in]
      }
      event Panel Close? {
        # "Send the 'Confirm Quit' message if the user closes the panel of the VI. Discard the event so the 'Confirm Quit' message has a chance to run."
        n187 = event-data() -> ()  [unwired: 1 in, 1 out]
        n188 = call-poly "Enqueue Message.vi"("Priority Message? (F)"=TRUE, "error in (no error)"=w520, "Message Data"="Are you sure?", "Message"="Confirm Quit", "Message Queue"=w523) -> ("error out"=w522:errorcluster, "dup Message Queue"=w521:refnum<queue>)  [unwired: 5 in]
        n189 = event-data("Discard?"=TRUE) -> ()  [unwired: 1 in, 1 out]
      }
      event Application Instance Close {
        # "#CodeRecommended - When a project closes, all VIs within that project are aborted and leave memory. However, any code placed in this event frame is guaranteed to run to completion, so add any cleanup code that absolutely must happen here."
        n190 = event-data() -> ()  [unwired: 1 in, 1 out]
      }
      event "Exit Button": Value Change {
        n191 = event-data() -> ()  [unwired: 1 in, 1 out]
        n192 = call-poly "Enqueue Message.vi"("Priority Message? Array"=bool[] [TRUE, TRUE], "error in (no error)"=w530, "Message Array"=string[] ["Turn Off Indicators", "Exit"], "Message Queue"=w532) -> ("error out"=w529:errorcluster, "dup Message Queue"=w531:refnum<queue>)  [unwired: 6 in]
      }
      event User Event {
        # "The Message Handling Loop processed an \"Exit\" message, which fired this event to stop the Event Handling Loop."
        n193 = event-data() -> ()  [unwired: 1 in, 1 out]
        n194 = local write "Display <Replace Me>"("\"Exit\" button pressed" ("VI Stopped")) -> ()
      }
    }
    n195 = call "Error Handler - Event Handling Loop.vi"("error in (no error)"=w503, "Message Queue"=w501) -> ("dup error in"=w500:errorcluster)  [unwired: 8 in, 1 out]
    n196 = Merge Errors(w500) -> (w499:errorcluster)
  }
  n197 = Unregister For Events(event registration refnum=w26, error in=w25) -> (error out=w27:errorcluster)
  n198 = Merge Errors(w21, w27, w23) -> (w19:errorcluster)
  n199 = call "close_visa_resources.vi"("error in (no error)"=w19, "VISA in"=w20) -> ("error out"=w14:errorcluster)  [unwired: 9 in]
  n200 = call <vilib>:"Destroy Rendezvous.vi"("error in (no error)"=w14, "rendezvous"=w8) -> ("error out"=w16:errorcluster)  [unwired: 4 in, 1 out]
  n201 = call "Destroy User Event - Stop.vi"("error in (no error)"=w16, "User Event - Stop"=w12) -> ("error out"=w15:errorcluster)  [unwired: 9 in]
  n202 = disable-structure shown="Default" {
    disable-tunnel: w15 -> [_ _]
    frame condition #0 (active) {
    }
    frame condition #1 {
      # "Call Quit LabVIEW if running as a built application."
      n203 = Quit LabVIEW() -> ()  [unwired: 1 in]
    }
  }
